vi "MetaJSONToListBox.vi"(8 "error in (no error)":errorcluster, 10 "JSON queue in":string, 11 "RefIn":refnum<vi>) -> (0 "error out":errorcluster)   [LabVIEW 2019]
uses:
  QueueControl.ctl
panel:
  # "Queue :"
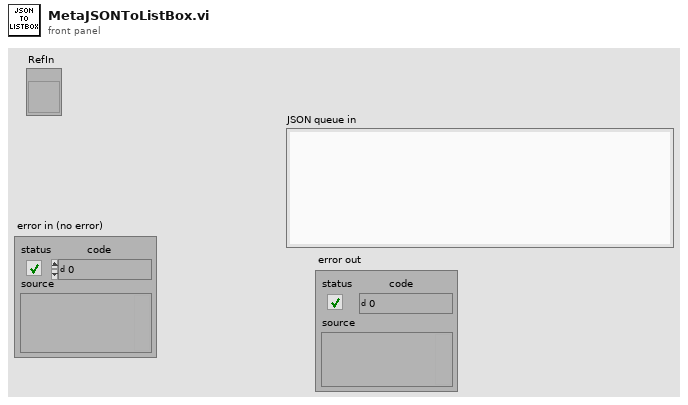
[diagram p1: front panel]
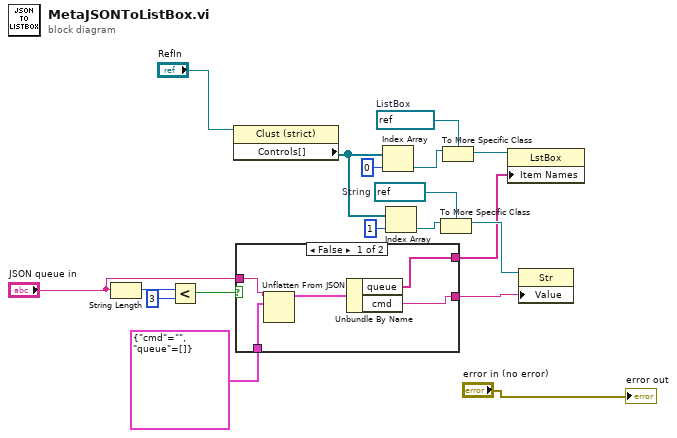
[diagram p0: block diagram]
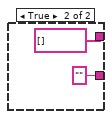
[diagram p2: hidden frame]
diagram:
  w11 = refnum<vi> refnum  # String
  w16 = refnum<vi> refnum  # ListBox
  n1 = String Length(string="JSON queue in") -> (length=w5:i32)
  n2 = Less?(x=w5, y=3) -> (x < y?=w3:bool)
  n3 = property class="Clust (strict)"(reference="RefIn") -> ("Controls[]"=w14:refnum<vi>[])  [unwired: 1 in, 2 out]
  n4 = case shown="False" w3 {
    tunnel: cluster{"cmd":string, "queue":string[]} {"cmd"="", "queue"=[]} -> [w23 _]
    tunnel: [w19 ""] -> w8
    tunnel: [w20 string[] [] ("queue")] -> w7
    tunnel: "JSON queue in" -> [w21 _]
    frame False {
      n5 = Unflatten From JSON(JSON string=w21, type and defaults=w23) -> (value=w22:cluster{"cmd":string, "queue":string[]})  [unwired: 5 in, 1 out]
      n6 = Unbundle By Name(w22) -> ("queue"=w20:string[], "cmd"=w19:string)
    }
    frame True {
    }
  }
  n7 = Index Array(array=w14, index=0) -> (element=w17:refnum<vi>)
  n8 = Index Array(array=w14, index=1) -> (element=w12:refnum<vi>)
  n9 = To More Specific Class(target class=w11, reference=w12) -> (specific class reference=w10:refnum<vi>)  [unwired: 1 in, 1 out]
  n10 = To More Specific Class(target class=w16, reference=w17) -> (specific class reference=w15:refnum<vi>)  [unwired: 1 in, 1 out]
  n11 = property class="LstBox"(reference=w15, "Item Names"=w7) -> ()  [unwired: 1 in, 2 out]
  n12 = property class="Str"(reference=w10, "Value"=w8) -> ()  [unwired: 1 in, 2 out]
  "error out" <- "error in (no error)"
